vi "BCtr2.vi"() -> ()   [LabVIEW 2015]
uses:
  <vilib>/Instr/_visa.llb/VISA Configure Serial Port (Instr).vi
panel:
  out "EOS":bool
  in  "StartIdx":i32
  in  "StrIn":string="M123mabcU3"
  out "Err":bool
  out "Idx":dbl
  out "error out":errorcluster
  out "Value":dbl
  out "Mode":string
  out "Modes":string[](array[string])
  out "Values":dbl[](array[numeric])
  out "Waveform Chart":u32(graph)
  out "Init":bool
  out "Reset":bool
  in  "Enable":bool
  in  "NB":u16[](array[numeric])
  in  "NA":u16[](array[numeric])
  in  "NC":u32 max=16777215 step=1
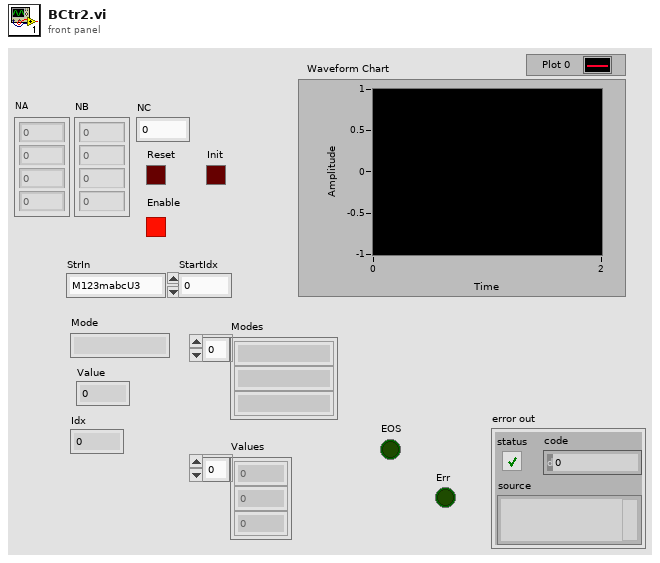
[diagram p1: front panel]
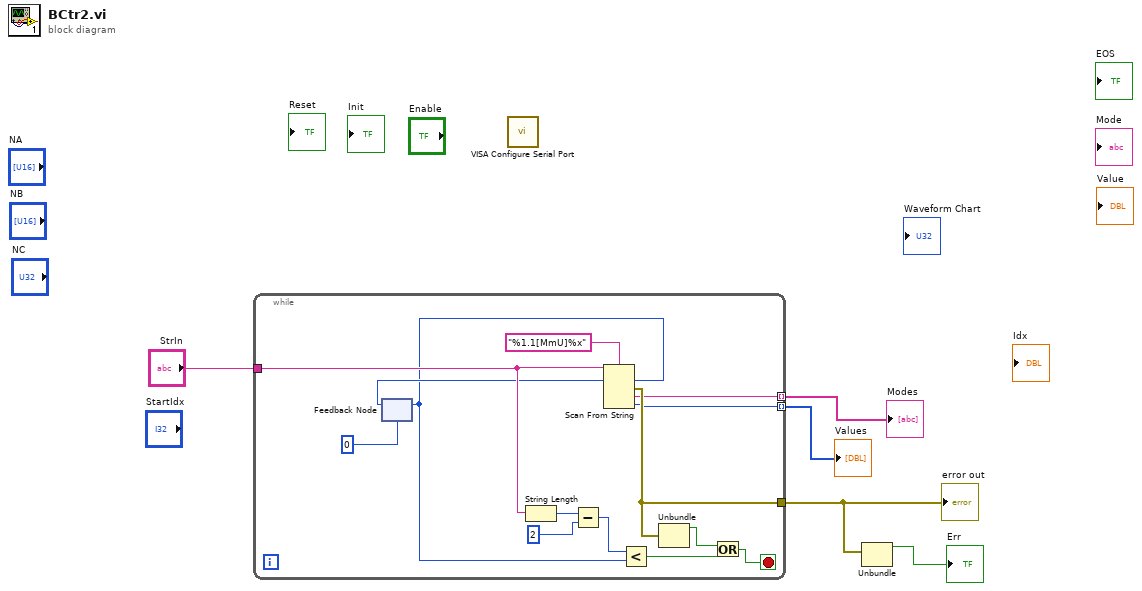
[diagram p0: block diagram]
diagram:
  n1 = while {
    tunnel: [w18] -> w4
    tunnel: "StrIn" -> [w14]
    tunnel: [w10] -> w2 mode=indexing
    tunnel: [w9] -> w1 mode=indexing
    stop <- w11 stop-if-true
    n2 = feedback #1(0) -> (w7:u32)
    n3 = String Length(string=w14) -> (length=w17:i32)
    n4 = Subtract(x=w17, y=2) -> (x-y=w15:i32)
    n5 = Scan From String(format string="%1.1[MmU]%x", input string=w14, initial scan location=w7) -> (offset past scan=w6:u32, error out=w18:errorcluster, output 1=w10:string, output 2=w9:u32)  [unwired: 3 in, 1 out]
    n6 = feedback-in #1(w6) -> ()
    n7 = Less?(x=w15, y=w6) -> (x < y?=w12:bool)
    n8 = Unbundle(w18) -> ("status"=w13:bool)  [unwired: 2 out]
    n9 = Or(x=w13, y=w12) -> (x .or. y?=w11:bool)
  }
  "Values" <- w1
  "Modes" <- w2
  "error out" <- w4
  n10 = call-poly "VISA Configure Serial Port"() -> ()  [unwired: 14 in, 2 out]
  n11 = Unbundle(w4) -> ("status"=→"Err":bool)  [unwired: 2 out]
